vi "Initialize CVT.vi"(8 "error in":errorcluster, 11 "Controller in":refnum<class "Controller.lvclass">) -> (0 "error out":errorcluster, 3 "Controller out":refnum<class "Controller.lvclass">)   [LabVIEW 2014, in "Controller.lvlib" / "Controller.lvclass"]
uses:
  Controller.lvclass
  SuperActor/SuperActor.lvclass/SuperActor.ctl
  SuperActor/Read CVT Session.vi
  SuperActor/Get Config Ref.vi
  <vilib>/Utility/config.llb/Read Key (String).vi
  <vilib>/Utility/config.llb/Read Key (Double).vi
  <vilib>/Utility/config.llb/Read Key (Boolean).vi
  SuperActor/SuperActor.lvclass
  <userlib>/_Session Fwk/Session - Root.lvclass
  <vilib>/Utility/config.llb/NI_LVConfig.lvlib
  reusable/Session APIs/CVT/CVT.lvclass
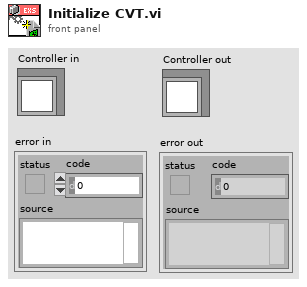
[diagram p1: front panel]
types:
  T1 = typedef "NI_LVConfig.lvlib/Config Data RefNum.ctl" = refnum<k1>
  T2 = typedef "Session - Root.lvclass/Session Handle.ctl" = refnum<data-value>
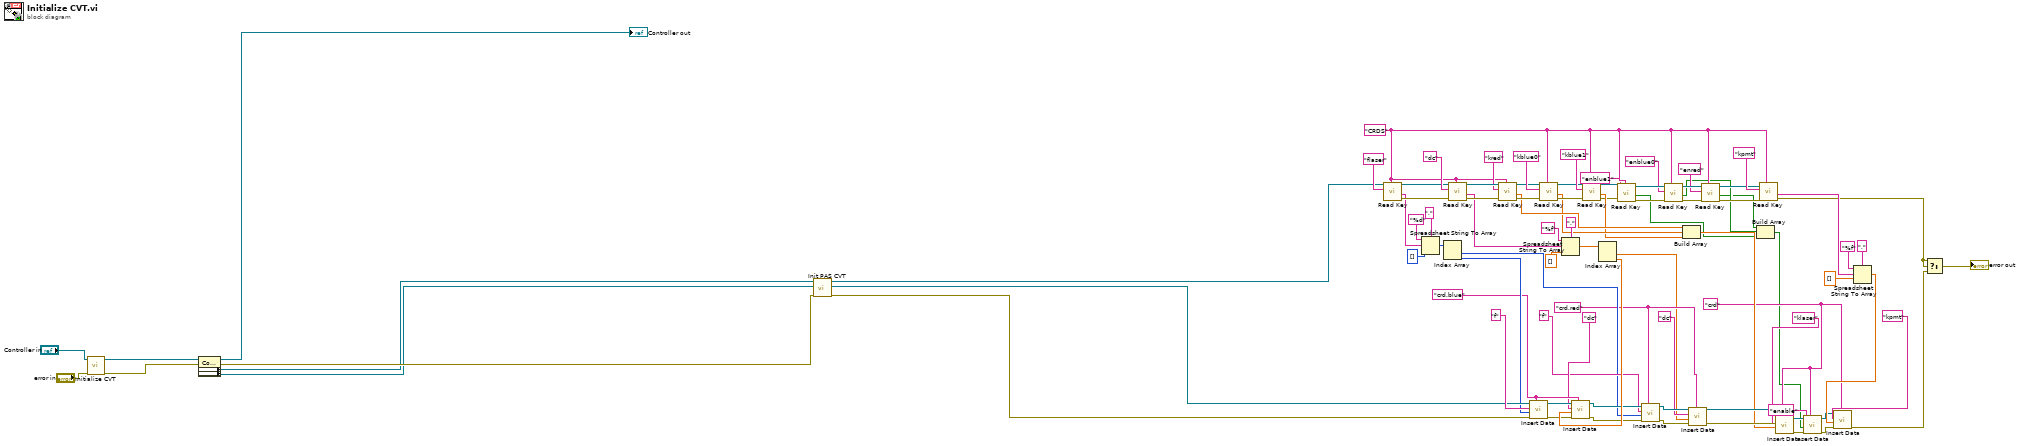
[diagram p0: block diagram]
diagram:
  w47 = "crd.blue" ("Group")
  w37 = "crd.red" ("Group")
  w3 = "crd" ("Group")
  w21 = "CRDS" ("section")
  n1 = call-parent "Initialize CVT.vi"("error in"="error in", "Ex Nested in"="Controller in") -> ("error out"=w27:errorcluster, "Ex Nested out"=w85:refnum<class "Controller.lvclass">)  [unwired: 8 in]
  n2 = property class="Controller"(reference=w85, error in=w27) -> (reference out=→"Controller out":refnum<class "Controller.lvclass">, error out=w87:errorcluster, "Config Ref"=w86:T1, "Accessors:CVT Session"=w84:T2)
  n3 = call "Init PAS CVT.vi"("error in"=w87, "CVT Session in"=w84, "Cfg Ref in"=w86) -> ("error out"=w49:errorcluster, "CVT Session Out"=w51:T2, "Refnum out"=w53:T1)  [unwired: 6 in]
  n4 = call-poly <vilib>:"Read Key.vi"("section"=w21, "key"="flaser", "refnum"=w53) -> ("error out"=w68:errorcluster, "value"=w58:string, "refnum out"=w67:T1)  [unwired: 5 in, 1 out]
  n5 = Spreadsheet String To Array(delimiter (Tab)=",", format string="%d", spreadsheet string=w58, array type (2D Dbl)=i16[] []) -> (array=w61:i16[])
  n6 = Index Array(array=w61) -> (element #1=w40:i16, element #2=w50:i16)  [unwired: 2 in]
  n7 = call-poly <vilib>:"Read Key.vi"("section"=w21, "error in (no error)"=w68, "key"="dc", "refnum"=w67) -> ("error out"=w74:errorcluster, "value"=w72:string, "refnum out"=w73:T1)  [unwired: 4 in, 1 out]
  n8 = call-poly <vilib>:"Read Key.vi"("section"=w21, "error in (no error)"=w74, "key"="kred" ("section"), "refnum"=w73) -> ("error out"=w77:errorcluster, "value"=w26:dbl, "refnum out"=w76:T1)  [unwired: 4 in, 1 out]
  n9 = call "Insert Data.vi"("Group"=w47, "error in"=w49, "Data"=w50, "tag"="f" ("Tag Name"), "CVT Session In"=w51) -> ("error out"=w44:errorcluster, "CVT Session Out"=w48:T2)  [unwired: 5 in]
  n10 = call-poly <vilib>:"Read Key.vi"("section"=w21, "error in (no error)"=w77, "key"="kblue0", "refnum"=w76) -> ("error out"=w79:errorcluster, "value"=w25:dbl, "refnum out"=w78:T1)  [unwired: 4 in, 1 out]
  n11 = Spreadsheet String To Array(delimiter (Tab)=",", format string="%f", spreadsheet string=w72, array type (2D Dbl)=sgl[] []) -> (array=w75:sgl[])
  n12 = call-poly <vilib>:"Read Key.vi"("section"=w21, "error in (no error)"=w79, "key"="kblue1", "refnum"=w78) -> ("error out"=w16:errorcluster, "value"=w24:dbl, "refnum out"=w20:T1)  [unwired: 4 in, 1 out]
  n13 = Index Array(array=w75) -> (element #1=w35:sgl, element #2=w45:sgl)  [unwired: 2 in]
  n14 = call "Insert Data.vi"("Group"=w47, "error in"=w44, "Data"=w45, "tag"="dc", "CVT Session In"=w48) -> ("error out"=w42:errorcluster, "CVT Session Out"=w43:T2)  [unwired: 5 in]
  n15 = call-poly <vilib>:"Read Key.vi"("section"=w21, "error in (no error)"=w16, "key"="enblue1", "refnum"=w20) -> ("error out"=w17:errorcluster, "value"=w10:bool, "refnum out"=w22:T1)  [unwired: 4 in, 1 out]
  n16 = call "Insert Data.vi"("Group"=w37, "error in"=w42, "Data"=w40, "tag"="f" ("Tag Name"), "CVT Session In"=w43) -> ("error out"=w38:errorcluster, "CVT Session Out"=w39:T2)  [unwired: 5 in]
  n17 = call-poly <vilib>:"Read Key.vi"("section"=w21, "error in (no error)"=w17, "key"="enblue0", "refnum"=w22) -> ("error out"=w18:errorcluster, "value"=w9:bool, "refnum out"=w19:T1)  [unwired: 4 in, 1 out]
  n18 = Build Array(w26, w25, w24) -> (w23:dbl[])
  n19 = call "Insert Data.vi"("Group"=w37, "error in"=w38, "Data"=w35, "tag"="dc", "CVT Session In"=w39) -> ("error out"=w33:errorcluster, "CVT Session Out"=w34:T2)  [unwired: 5 in]
  n20 = call-poly <vilib>:"Read Key.vi"("section"=w21, "error in (no error)"=w18, "key"="enred", "refnum"=w19) -> ("error out"=w12:errorcluster, "value"=w8:bool, "refnum out"=w13:T1)  [unwired: 4 in, 1 out]
  n21 = Build Array(w8, w9, w10) -> (w1:bool[])
  n22 = call-poly <vilib>:"Read Key.vi"("section"=w21, "error in (no error)"=w12, "key"="kpmt" ("section"), "refnum"=w13) -> ("error out"=w29:errorcluster, "value"=w63:string)  [unwired: 4 in, 2 out]
  n23 = call "Insert Data.vi"("Group"=w3, "error in"=w33, "Data"=w23, "tag"="klaser", "CVT Session In"=w34) -> ("error out"=w6:errorcluster, "CVT Session Out"=w7:T2)  [unwired: 5 in]
  n24 = call "Insert Data.vi"("Group"=w3, "error in"=w6, "Data"=w1, "tag"="enable", "CVT Session In"=w7) -> ("error out"=w4:errorcluster, "CVT Session Out"=w5:T2)  [unwired: 5 in]
  n25 = Spreadsheet String To Array(delimiter (Tab)=",", format string="%f", spreadsheet string=w63, array type (2D Dbl)=sgl[] []) -> (array=w30:sgl[])
  n26 = call "Insert Data.vi"("Group"=w3, "error in"=w4, "Data"=w30, "tag"="kpmt" ("Tag Name"), "CVT Session In"=w5) -> ("error out"=w28:errorcluster)  [unwired: 5 in, 1 out]
  n27 = Select(t=w29, s=w29, f=w28) -> (s? t:f=→"error out":errorcluster)
